vi "Get or Create Instrument.vi"(8 "Error In":errorcluster, 10 "Instrument Identifier":string) -> (0 "Error Out":errorcluster, 2 "IInstrument":refnum<class "IInstrument.lvclass">)   [LabVIEW 2024, in "Instrument Manager.lvclass"]
uses:
  Instrument Manager.lvclass
  Interfaces/IInstrument/IInstrument.lvclass
  Interfaces/IConfigurable/IConfigurable.lvclass
  Instrument Manager.lvclass/Instrument Manager.ctl
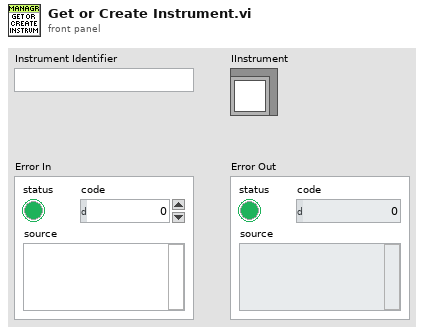
[diagram p1: front panel]
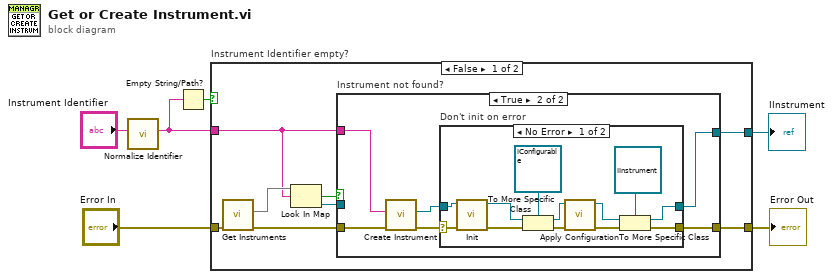
[diagram p0: block diagram]
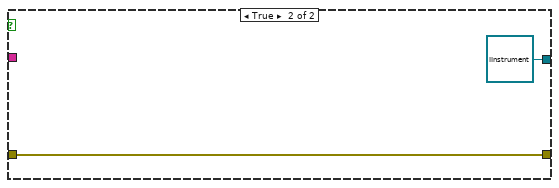
[diagram p4: hidden frame]
diagram:
  n1 = call "Normalize Identifier.vi"("Identifier"="Instrument Identifier") -> ("Normalized Identifier"=w1:string)  [unwired: 10 in]
  n2 = Empty String/Path?(string/path=w1) -> (empty?=w2:bool)
  n3 = case "Instrument Identifier empty?" shown="False" w2 {
    tunnel: [w14 w37] -> w6
    tunnel: [w13 refnum<class "IInstrument.lvclass"> refnum ("IInstrument out")] -> w5
    tunnel: "Error In" -> [w12 w37]
    tunnel: w1 -> [w7 _]
    frame False {
      n4 = call "Get Instruments.vi"("Error In"=w12) -> ("Error Out"=w11:errorcluster, "IInstruments"=w10:map{string, refnum<class "IInstrument.lvclass">})  [unwired: 9 in]
      n5 = Look In Map(map=w10, key=w7) -> (key not found?=w9:bool, value=w8:refnum<class "IInstrument.lvclass">)  [unwired: 1 in]
      n6 = case "Instrument not found?" shown="True" w9 {
        tunnel: [w15 w20] -> w14
        tunnel: w11 -> [w15 w21]
        tunnel: w8 -> [w16 _]
        tunnel: [w16 w19] -> w13
        tunnel: w7 -> [_ w18]
        frame False {
        }
        frame True {
          n7 = call "Create Instrument.vi"("error in"=w21, "Instrument Identifier"=w18) -> ("error out"=w22:errorcluster, "IInstrument out"=w17:refnum<class "IInstrument.lvclass">)  [unwired: 8 in]
          n8 = case "Don't init on error" shown="No Error" w22 {
            selector: w22 -> [w34 w36]
            tunnel: [w28 w36] -> w20
            tunnel: [w26 w35] -> w19
            tunnel: w17 -> [w23 w35]
            frame No Error {
              n9 = call-dynamic "Init.vi"("error in"=w34, "IInitialize in"=w23) -> ("error out"=w33:errorcluster, "IInitialize out"=w25:refnum<class "IInstrument.lvclass">)  [unwired: 8 in]
              n10 = To More Specific Class(target class=refnum<class "IConfigurable.lvclass"> refnum ("IConfigurable.lvclass"), reference=w25, error in=w33) -> (specific class reference=w29:refnum<class "IConfigurable.lvclass">, error out=w31:errorcluster)
              n11 = call-dynamic "Apply Configuration.vi"("error in"=w31, "IConfigurable in"=w29) -> ("error out"=w32:errorcluster, "IConfigurable out"=w27:refnum<class "IConfigurable.lvclass">)  [unwired: 8 in]
              n12 = To More Specific Class(target class=refnum<class "IInstrument.lvclass"> refnum ("IInstrument.lvclass"), reference=w27, error in=w32) -> (specific class reference=w26:refnum<class "IInstrument.lvclass">, error out=w28:errorcluster)
            }
            frame Error {
            }
          }
        }
      }
    }
    frame True {
    }
  }
  "Error Out" <- w6
  "IInstrument" <- w5
